vi "Set_And_Save_Init.vi"(0 "Filename (.ini)":string="pulse_sequence_default.ini", 1 "error in":errorcluster) -> (2 "Init outp register 1 (2-7)":bool[](array[boolean]), 3 "Init outp register 2 (8-13)":bool[](array[boolean]), 4 "error out":errorcluster)   [LabVIEW 2021]
uses:
  Pulse_Sequence_Global.vi
  <vilib>/Utility/config.llb/Write Key (Boolean).vi
  <vilib>/Utility/config.llb/NI_LVConfig.lvlib
panel:
  # "Remember that config files are .ini, \nconfig file will be save in ...\\Config_Files\\(filename).ini"
  # "All used channels should be specified here"
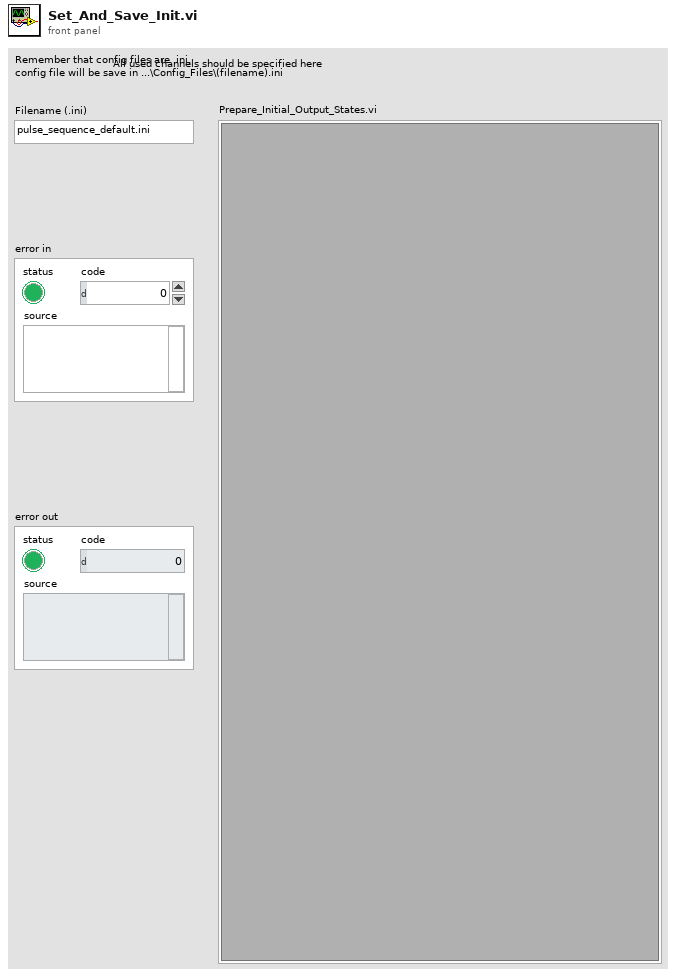
[diagram p1: front panel]
types:
  T1 = typedef "NI_LVConfig.lvlib/Config Data RefNum.ctl" = refnum<k1>
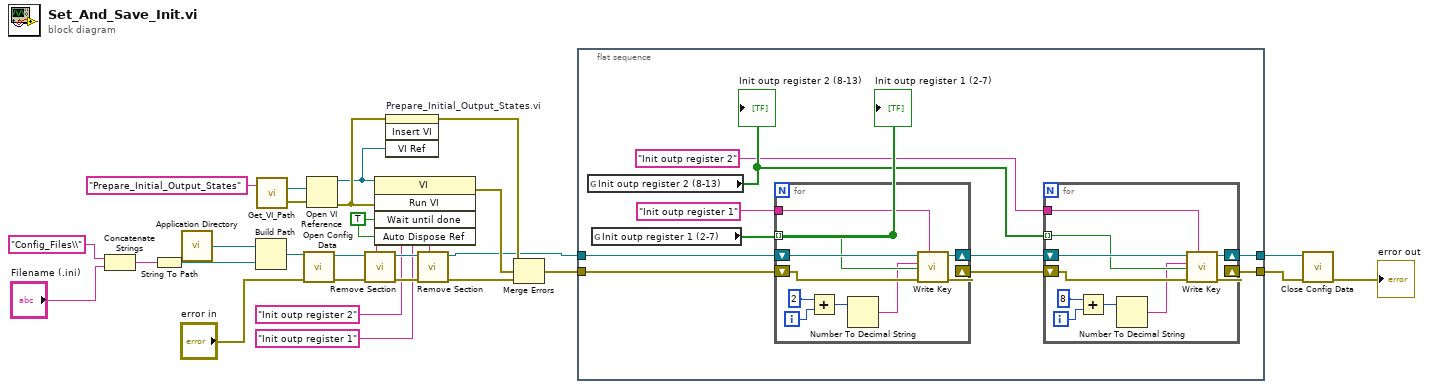
[diagram p0: block diagram]
diagram:
  w21 = TRUE ("Wait Until Done")
  n1 = Concatenate Strings("Config_Files\\" ("string"), "Filename (.ini)") -> (w13:string)
  n2 = String To Path(string=w13) -> (path=w19:path)
  n3 = call <vilib>:"Application Directory.vi"() -> ("Application Directory"=w27:path)
  n4 = Build Path(base path=w27, name or relative path=w19) -> (appended path=w26:path)
  n5 = call "Get_VI_Path.vi"("VI name (no .vi)"="Prepare_Initial_Output_States") -> ("error out"=w22:errorcluster, "File Path"=w24:path)  [unwired: 1 in]
  n6 = call <vilib>:"Open Config Data.vi"("error in (no error)"="error in", "configuration file path"=w26) -> ("error out"=w5:errorcluster, "refnum"=w7:T1)  [unwired: 7 in, 1 out]
  n7 = Open VI Reference(vi path=w24, error in (no error)=w22) -> (vi reference=w1:refnum<vi>, error out=w20:errorcluster)  [unwired: 4 in]
  n8 = call <vilib>:"Remove Section.vi"("section"="Init outp register 2", "error in (no error)"=w5, "refnum"=w7) -> ("error out"=w9:errorcluster, "refnum out"=w8:T1)  [unwired: 6 in, 1 out]
  n9 = invoke class="VI" method="Run VI"(reference=w1, error in=w20, "Wait until done"=w21, "Auto Dispose Ref"=w21) -> (error out=w18:errorcluster)  [unwired: 1 in, 4 out]
  n10 = invoke on="Prepare_Initial_Output_States.vi" class="SubPnl" method="Insert VI"(error in=w20, "VI Ref"=w1) -> (error out=w17:errorcluster)  [unwired: 2 in, 3 out]
  n11 = call <vilib>:"Remove Section.vi"("section"="Init outp register 1", "error in (no error)"=w9, "refnum"=w8) -> ("error out"=w4:errorcluster, "refnum out"=w6:T1)  [unwired: 6 in, 1 out]
  n12 = Merge Errors(w17, w18, w4) -> (w16:errorcluster)
  n13 = flat-sequence {
    tunnel: w16 -> [w37]
    tunnel: w6 -> [w36]
    tunnel: [w29] -> w12
    tunnel: [w28] -> w11
    frame #0 {
      n14 = global read "Pulse_Sequence_Global.vi" "Init outp register 2 (8-13)"() -> (w31:bool[])
      "Init outp register 2 (8-13)" <- w31
      n15 = global read "Pulse_Sequence_Global.vi" "Init outp register 1 (2-7)"() -> (w35:bool[])
      "Init outp register 1 (2-7)" <- w35
      n16 = for {
        tunnel: w35 -> [w51] mode=indexing
        shift-right: [w56] -> w33
        shift-left: w37 -> [w54]
        shift-right: [w55] -> w32
        shift-left: w36 -> [w57]
        tunnel: "Init outp register 1" ("section") -> [w48]
        i -> [w53]
        n17 = Add(x=2, y=w53) -> (x+y=w50:i32)
        n18 = Number To Decimal String(number=w50) -> (decimal integer string=w49:string)  [unwired: 1 in]
        n19 = call-poly <vilib>:"Write Key.vi"("section"=w48, "error in (no error)"=w54, "value"=w51, "key"=w49, "refnum"=w57) -> ("error out"=w56:errorcluster, "refnum out"=w55:T1)  [unwired: 4 in, 1 out]
      }
      n20 = for {
        tunnel: w31 -> [w41] mode=indexing
        shift-right: [w46] -> w29
        shift-left: w33 -> [w44]
        shift-right: [w45] -> w28
        shift-left: w32 -> [w47]
        tunnel: "Init outp register 2" ("section") -> [w38]
        i -> [w43]
        n21 = Add(x=8, y=w43) -> (x+y=w40:i32)
        n22 = Number To Decimal String(number=w40) -> (decimal integer string=w39:string)  [unwired: 1 in]
        n23 = call-poly <vilib>:"Write Key.vi"("section"=w38, "error in (no error)"=w44, "value"=w41, "key"=w39, "refnum"=w47) -> ("error out"=w46:errorcluster, "refnum out"=w45:T1)  [unwired: 4 in, 1 out]
      }
    }
  }
  n24 = call <vilib>:"Close Config Data.vi"("error in (no error)"=w12, "refnum"=w11) -> ("error out"=→"error out":errorcluster)  [unwired: 8 in, 1 out]
